vi "Set Relation.vi"(10 "Relation":T1, 11 "Base Sender in":refnum<class "Base Sender.lvclass">) -> (3 "Base Sender out":refnum<class "Base Sender.lvclass">)   [LabVIEW 2020, in "jettl.lvlib" / "Sender.lvlib" / "Base Sender.lvclass"]
uses:
  Base Sender.lvclass
  Relation.ctl
  Sender.lvlib
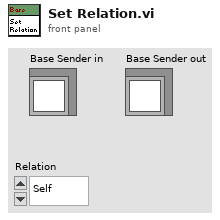
[diagram p1: front panel]
types:
  T1 = typedef "jettl.lvlib/Sender.lvlib/Relation.ctl" = enum16{"Self", "Creator", "Created"}
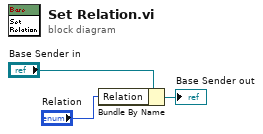
[diagram p0: block diagram]
diagram:
  n1 = Bundle By Name(cluster="Base Sender in", "Relation"="Relation") -> (→"Base Sender out":refnum<class "Base Sender.lvclass">)
